vi "Expt9_MT Spread-Despread_Student_lab.vi"() -> ()   [LabVIEW 2020]
doc: "This example demonstrates spreading and despreading."
uses:
  <vilib>/addons/Modulation/Digital/General/MT Generate Bits (Galois, PN Order).vi
  <vilib>/addons/Modulation/niDMT.lvlib
  <vilib>/addons/Modulation/Digital/General/MT Generate Bits (User Defined).vi
  <vilib>/Utility/file.llb/Read Delimited Spreadsheet (DBL).vi
panel:
  in  "Spreading Sequence Length":i32=4
  in  "PN Sequence Order (Message)":i32=9
  in  "Spreading Sequence Type":T1(tab)
  in  "PN Sequence Order":i32=9
  in  "User Base Bit Pattern":i8[](array[numeric])=[1, 0, 1, 1, 0, 1]
  in  "Path":path
  out "Error Out":errorcluster
  out "Encoded Bit Count":i32
  out "Noise":i8[](array[numeric])
  out "Bit Error Rate":dbl
  in  "Noise (bit flip probability)":dbl=0.03 format="%.6g"
  out "Message Bits":i8[](array[numeric])
  out "Spread Bits":i8[](array[numeric])
  out "Despread Bits":i8[](array[numeric])
  in  "Message Bits":i32=1000
  # "Spread/Despread Programming Example"
  # "File format : 1 bit per line"
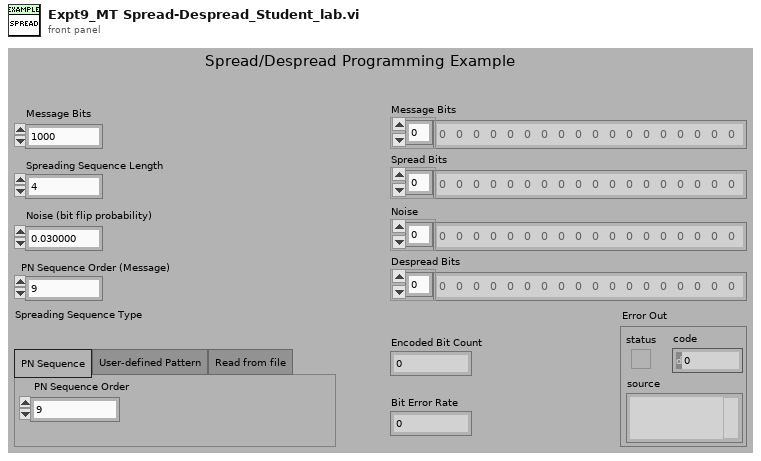
[diagram p1: front panel]
types:
  T1 = enum32{"PN Sequence", "User-defined Pattern", "Read from file"}
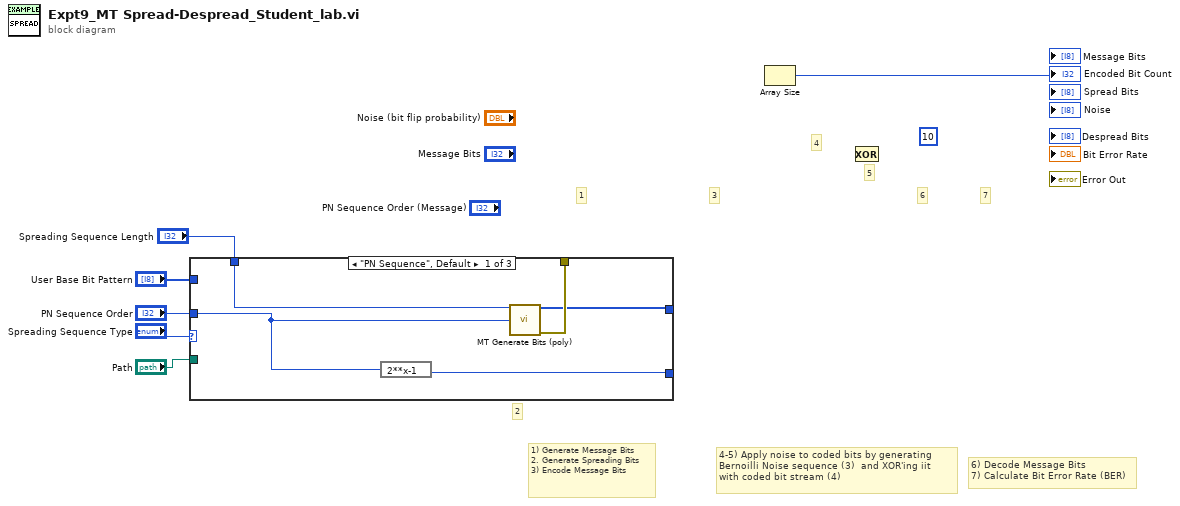
[diagram p0: block diagram]
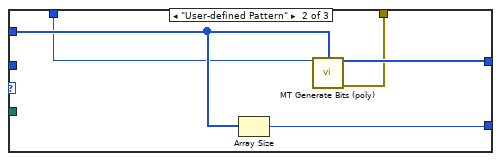
[diagram p2: hidden frame]
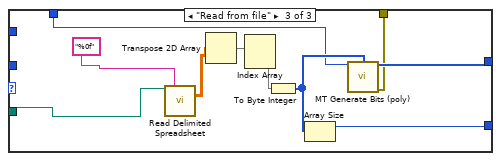
[diagram p3: hidden frame]
diagram:
  (unwired) 10 ("sync search depth (bits)")
  # "2"
  # "7"
  # "6"
  # "5"
  # "4"
  # "3"
  # "1"
  # "6) Decode Message Bits\n7) Calculate Bit Error Rate (BER)"
  # "1) Generate Message Bits\n2. Generate Spreading Bits\n3) Encode Message Bits"
  # "4-5) Apply noise to coded bits by generating \nBernoilli Noise sequence (3)  and XOR'ing iit \nwith coded bit stream (4)"
  n1 = case shown="\"PN Sequence\", Default" "Spreading Sequence Type" {
    tunnel: "User Base Bit Pattern" -> [_ w15 _]
    tunnel: [w7 w13 w21] -> _
    tunnel: [w11 w16 w24] -> _
    tunnel: "PN Sequence Order" -> [w9 _ _]
    tunnel: "Path" -> [_ _ w17]
    tunnel: "Spreading Sequence Length" -> [w10 w14 w22]
    tunnel: [w8 w12 w20] -> _
    frame "PN Sequence", Default {
      n2 = expression code="2**x-1"(w9) -> (w11:i32)
      n3 = call-poly <vilib>:"MT Generate Bits (poly).vi"("total bits (128)"=w10, "PN sequence order (9)"=w9) -> ("output bit stream"=w7:i8[], "error out"=w8:errorcluster)  [unwired: 11 in, 1 out]
    }
    frame "User-defined Pattern" {
      n4 = Array Size(array=w15) -> (size(s)=w16:i32)
      n5 = call-poly <vilib>:"MT Generate Bits (poly).vi"("total bits (128)"=w14, "user base bit pattern"=w15) -> ("output bit stream"=w13:i8[], "error out"=w12:errorcluster)  [unwired: 12 in]
    }
    frame "Read from file" {
      n6 = call-poly <vilib>:"Read Delimited Spreadsheet.vi"("file path (dialog if empty)"=w17, "format (%.3f)"="%0f") -> ("all rows"=w19:dbl[][])  [unwired: 8 in, 5 out]
      n7 = Transpose 2D Array(2D array=w19) -> (transposed array=w25:dbl[][])
      n8 = Index Array(array=w25) -> (element=w26:dbl[])  [unwired: 2 in]
      n9 = To Byte Integer(number=w26) -> (8bit integer=w23:i8[])
      n10 = Array Size(array=w23) -> (size(s)=w24:i32)
      n11 = call-poly <vilib>:"MT Generate Bits (poly).vi"("total bits (128)"=w22, "user base bit pattern"=w23) -> ("output bit stream"=w21:i8[], "error out"=w20:errorcluster)  [unwired: 12 in]
    }
  }
  n12 = Array Size() -> (size(s)=→"Encoded Bit Count":i32)  [unwired: 1 in]
  n13 = Exclusive Or() -> ()  [unwired: 2 in, 1 out]
